vi "Read position.vi"(11 "RelayInterface in":refnum<class "RelayInterface.lvclass">) -> (2 "position":T1=10 items=["Open"=10, "Closed"=11], 3 "RelayInterface out":refnum<class "RelayInterface.lvclass">)   [LabVIEW 2015, in "SLSC Switch.lvlib" / "RelayInterface.lvclass"]
doc: "This reads the position of a relay"
uses:
  RelayInterface.lvclass
  slscsl/RelayPosition.ctl
  RelayInterface.lvclass/RelayInterface.ctl
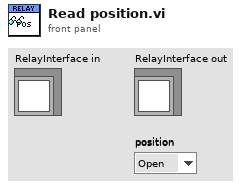
[diagram p1: front panel]
types:
  T1 = typedef "SLSC Switch.lvlib/slscsl.lvclass/RelayPosition.ctl" = i32
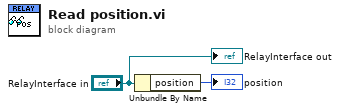
[diagram p0: block diagram]
diagram:
  n1 = Unbundle By Name("RelayInterface in") -> ("position"=→"position":T1)
  "RelayInterface out" <- "RelayInterface in"
